vi "input.vi"(8 "error in":errorcluster, 10 "data table in":T1, 11 "OPC UA runtime in":refnum<class "OPC UA Server runtime.lvclass">) -> (0 "error out":errorcluster, 2 "data table out":T1, 3 "OPC UA runtime out":refnum<class "OPC UA Server runtime.lvclass">)   [LabVIEW 2013, in "OPC UA Server runtime.lvclass"]
doc: "Provides an interface for reading data from a module at runtime. While this interface performs no operations, a child should provide an override which may read from any open sessions, references, or interfaces."
uses:
  OPC UA Server runtime.lvclass
  <vilib>/NI/Tag Bus/table/data table.ctl
  OPC UA Server runtime.lvclass/OPC UA Server runtime.ctl
  <vilib>/NI/Tag Bus/table/data polymorphs/write one/write Boolean.vi
  <vilib>/NI/Tag Bus/table/data polymorphs/write one/write I8.vi
  <vilib>/NI/Tag Bus/table/data polymorphs/write one/write U8.vi
  <vilib>/NI/Tag Bus/table/data polymorphs/write one/write I16.vi
  <vilib>/NI/Tag Bus/table/data polymorphs/write one/write U16.vi
  <vilib>/NI/Tag Bus/table/data polymorphs/write one/write I32.vi
  <vilib>/NI/Tag Bus/table/data polymorphs/write one/write U32.vi
  <vilib>/NI/Tag Bus/table/data polymorphs/write one/write I64.vi
  <vilib>/NI/Tag Bus/table/data polymorphs/write one/write U64.vi
  <vilib>/NI/Tag Bus/table/data polymorphs/write one/write Single.vi
  <vilib>/NI/Tag Bus/table/data polymorphs/write one/write Double.vi
  <vilib>/NI/Tag Bus/table/data polymorphs/write one/write String.vi
  <vilib>/NI/Tag Bus/table/data polymorphs/write one/write Array of Boolean.vi
  <vilib>/NI/Tag Bus/table/data polymorphs/write one/write Array of I8.vi
  <vilib>/NI/Tag Bus/table/data polymorphs/write one/write Array of U8.vi
  <vilib>/NI/Tag Bus/table/data polymorphs/write one/write Array of I16.vi
  <vilib>/NI/Tag Bus/table/data polymorphs/write one/write Array of U16.vi
  <vilib>/NI/Tag Bus/table/data polymorphs/write one/write Array of I32.vi
  <vilib>/NI/Tag Bus/table/data polymorphs/write one/write Array of U32.vi
  <vilib>/NI/Tag Bus/table/data polymorphs/write one/write Array of I64.vi
  <vilib>/NI/Tag Bus/table/data polymorphs/write one/write Array of U64.vi
  <vilib>/NI/Tag Bus/table/data polymorphs/write one/write Array of Single.vi
  <vilib>/NI/Tag Bus/table/data polymorphs/write one/write Array of Double.vi
  <vilib>/NI/Tag Bus/table/data polymorphs/write one/write Array of String.vi
  <vilib>/OPCUA/server/Read Bool.vi
  <vilib>/OPCUA/server/Read SByte.vi
  <vilib>/OPCUA/server/Read Byte.vi
  <vilib>/OPCUA/server/Read Int16.vi
  <vilib>/OPCUA/server/Read UInt16.vi
  <vilib>/OPCUA/server/Read Int32.vi
  <vilib>/OPCUA/server/Read UInt32.vi
  <vilib>/OPCUA/server/Read Int64.vi
  <vilib>/OPCUA/server/Read UInt64.vi
  <vilib>/OPCUA/server/Read Float.vi
  <vilib>/OPCUA/server/Read Double.vi
  <vilib>/OPCUA/server/Read String.vi
  <vilib>/OPCUA/server/Read Date Time.vi
  <vilib>/OPCUA/server/Read Byte String.vi
  <vilib>/OPCUA/server/Read Bool Array.vi
  <vilib>/OPCUA/server/Read SByte Array.vi
  <vilib>/OPCUA/server/Read Byte Array.vi
  <vilib>/OPCUA/server/Read Int16 Array.vi
  <vilib>/OPCUA/server/Read UInt16 Array.vi
  <vilib>/OPCUA/server/Read Int32 Array.vi
  <vilib>/OPCUA/server/Read UInt32 Array.vi
  <vilib>/OPCUA/server/Read Int64 Array.vi
  <vilib>/OPCUA/server/Read UInt64 Array.vi
  <vilib>/OPCUA/server/Read Float Array.vi
  <vilib>/OPCUA/server/Read Double Array.vi
  <vilib>/OPCUA/server/Read String Array.vi
  <vilib>/OPCUA/server/Read Date Time Array.vi
  <vilib>/OPCUA/server/Read Byte String Array.vi
  <vilib>/Utility/error.llb/Error Cluster From Error Code.vi
  <vilib>/OPCUA/client/Read Bool.vi
  <vilib>/OPCUA/client/Read SByte.vi
  <vilib>/OPCUA/client/Read Byte.vi
  <vilib>/OPCUA/client/Read Int16.vi
  <vilib>/OPCUA/client/Read UInt16.vi
  <vilib>/OPCUA/client/Read Int32.vi
  <vilib>/OPCUA/client/Read UInt32.vi
  <vilib>/OPCUA/client/Read Int64.vi
  <vilib>/OPCUA/client/Read UInt64.vi
  <vilib>/OPCUA/client/Read Float.vi
  <vilib>/OPCUA/client/Read Double.vi
  <vilib>/OPCUA/client/Read String.vi
  <vilib>/OPCUA/client/Read DateTime.vi
  <vilib>/OPCUA/client/Read ByteString.vi
  <vilib>/OPCUA/client/Read Bool Array.vi
  <vilib>/OPCUA/client/Read SByte Array.vi
  <vilib>/OPCUA/client/Read Byte Array.vi
  <vilib>/OPCUA/client/Read Int16 Array.vi
  <vilib>/OPCUA/client/Read UInt16 Array.vi
  <vilib>/OPCUA/client/Read Int32 Array.vi
  <vilib>/OPCUA/client/Read UInt32 Array.vi
  <vilib>/OPCUA/client/Read Int64 Array.vi
  <vilib>/OPCUA/client/Read UInt64 Array.vi
  <vilib>/OPCUA/client/Read Float Array.vi
  <vilib>/OPCUA/client/Read Double Array.vi
  <vilib>/OPCUA/client/Read String Array.vi
  <vilib>/OPCUA/client/Read DateTime Array.vi
  <vilib>/OPCUA/client/Read ByteString Array.vi
  <vilib>/ErrorRing/Error Ring.xnode
  <vilib>/NI/Tag Bus/table/data table.lvlib
  <vilib>/opcua/NI OPC UA Client.lvlib
  <vilib>/opcua/NI OPC UA Server.lvlib
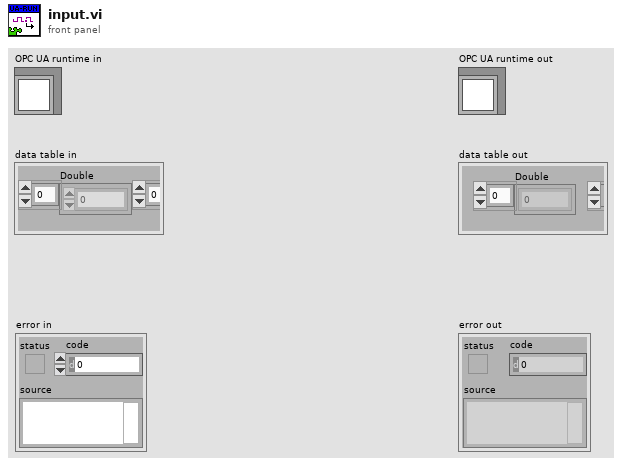
[diagram p1: front panel]
types:
  T1 = typedef "tag bus.lvlib/data table.lvlib/data table.ctl" = cluster{"Double":dbl[], "Single":sgl[], "I64":i64[], "I32":i32[], "I16":i16[], "I8":i8[], "U64":u64[], "U32":u32[], "U16":u16[], "U8":u8[], "Boolean":bool[], "String":string[], "Array of Double":cluster{"DBL Array":dbl[]}[], "Array of Single":cluster{"SGL Array":sgl[]}[], "Array of I64":cluster{"I64 Array":i64[]}[], "Array of I32":cluster{"I32 Array":i32[]}[], "Array of I16":cluster{"I16 Array":i16[]}[], "Array of I8":cluster{"I8 Array":i8[]}[], "Array of U64":cluster{"U64 Array":u64[]}[], "Array of U32":cluster{"U32 Array":u32[]}[], "Array of U16":cluster{"U16 Array":u16[]}[], "Array of U8":cluster{"U8 Array":u8[]}[], "Array of Boolean":cluster{"Boolean Array":bool[]}[], "Array of String":cluster{"String Array":string[]}[]}
  T2 = typedef "tag bus.lvlib/tag descriptor.lvclass/Data Type.ctl" = enum16{"Double", "Single", "I64", "I32", "I16", "I8", "U64", "U32", "U16", "U8", "Boolean", "String", "Array of Double", "Array of Single", "Array of I64", "Array of I32", "Array of I16", "Array of I8", "Array of U64", "Array of U32", "Array of U16", "Array of U8", "Array of Boolean", "Array of String"}
  T3 = typedef "OPC UA Server configuration.lvclass/OPC UA Data Type.ctl" = u16
  T4 = cluster{"DCAF Data Type":T2, "Index":i32, "Node Path":string, "OPC UA Data Type":T3}[]
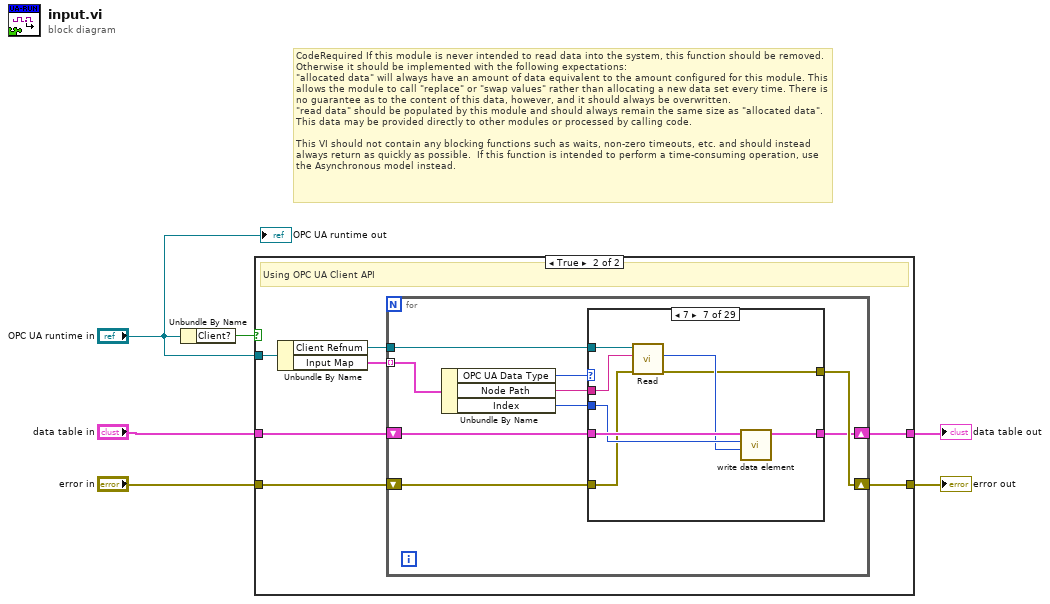
[diagram p0: block diagram]
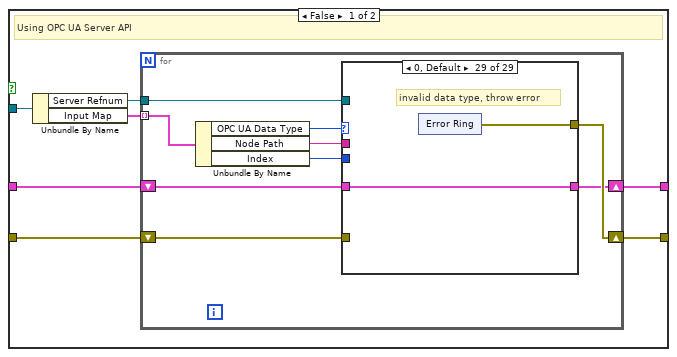
[diagram p2: hidden frame]
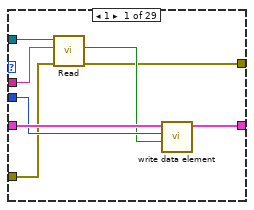
[diagram p3: hidden frame]
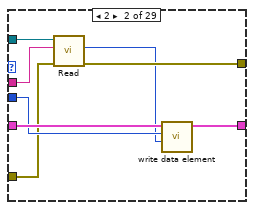
[diagram p4: hidden frame]
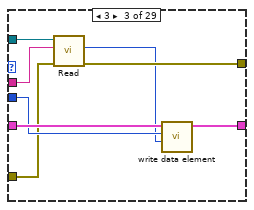
[diagram p5: hidden frame]
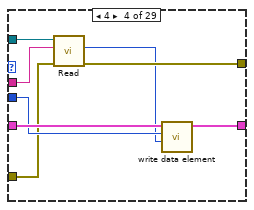
[diagram p6: hidden frame]
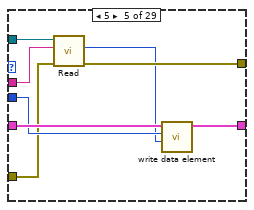
[diagram p7: hidden frame]
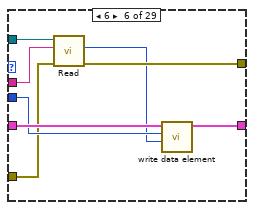
[diagram p8: hidden frame]
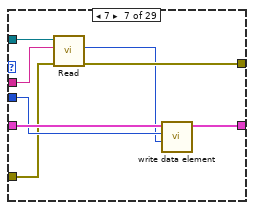
[diagram p9: hidden frame]
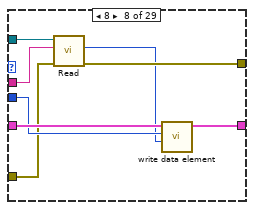
[diagram p10: hidden frame]
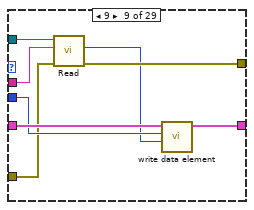
[diagram p11: hidden frame]
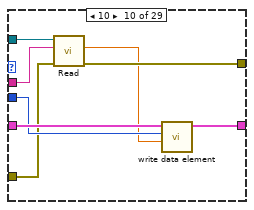
[diagram p12: hidden frame]
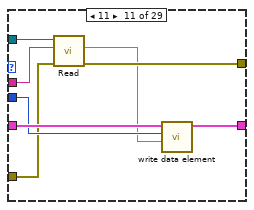
[diagram p13: hidden frame]
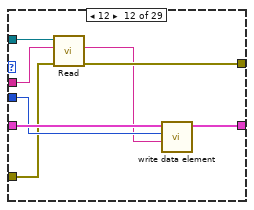
[diagram p14: hidden frame]
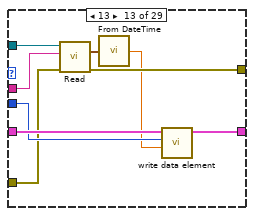
[diagram p15: hidden frame]
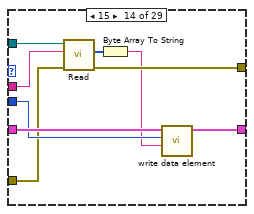
[diagram p16: hidden frame]
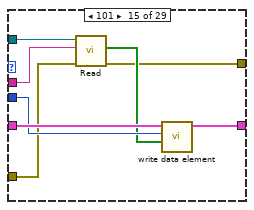
[diagram p17: hidden frame]
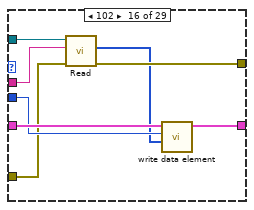
[diagram p18: hidden frame]
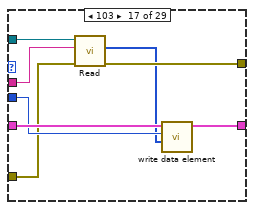
[diagram p19: hidden frame]
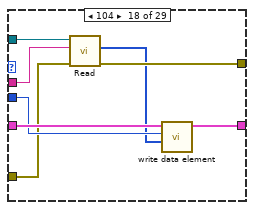
[diagram p20: hidden frame]
diagram:
  # "CodeRequired If this module is never intended to read data into the system, this function should be removed. Otherwise it should be implemented with the following expectations:\n\"allocated data\" will always have an amount of data equivalent to the amount configured for this module. This allows the module to call \"replace\" or \"swap values\" rather than allocating a new data set every time. There is no guarantee as to the content of this data, however, and it should always be overwritten.\n\"read data\" should be populated by this module and should always remain the same size as \"allocated data\". This data may be provided directly to other modules or processed by calling code.\n\nThis VI should not contain any blocking functions such as waits, non-zero timeouts, etc. and should instead always return as quickly as possible.  If this function is intended to perform a time-consuming operation, use the Asynchronous model instead."
  n1 = Unbundle By Name("OPC UA runtime in") -> ("Client?"=w6:bool)
  n2 = case shown="True" w6 {
    tunnel: "OPC UA runtime in" -> [w13 w266]
    tunnel: "data table in" -> [w9 w263]
    tunnel: "error in" -> [w8 w262]
    tunnel: [w10 w261] -> w2
    tunnel: [w7 w260] -> w1
    frame False {
      # "Using OPC UA Server API"
      n3 = Unbundle By Name(w13) -> ("Server Refnum"=w11:refnum<k21>, "Input Map"=w12:T4)
      n4 = for {
        tunnel: w11 -> [w18]
        tunnel: w12 -> [w22] mode=indexing
        shift-right: [w15] -> w7
        shift-left: w8 -> [w16]
        shift-right: [w14] -> w10
        shift-left: w9 -> [w17]
        n5 = Unbundle By Name(w22) -> ("OPC UA Data Type"=w21:T3, "Node Path"=w20:string, "Index"=w19:i32)
        n6 = case shown="0, Default" w21 {
          tunnel: w20 -> [w29 w37 w45 w53 w61 w69 w77 w85 w93 w101 w109 w117 w126 w135 w144 w152 w160 w168 w176 w184 w192 w200 w208 w216 w224 w232 w241 w249 _]
          tunnel: w19 -> [w27 w35 w43 w51 w59 w67 w75 w83 w91 w99 w107 w115 w124 w133 w142 w150 w158 w166 w174 w182 w190 w198 w206 w214 w222 w230 w239 w247 _]
          tunnel: w18 -> [w30 w38 w46 w54 w62 w70 w78 w86 w94 w102 w110 w118 w127 w136 w137 w146 w153 w162 w170 w178 w186 w194 w202 w210 w218 w225 w234 w250 _]
          tunnel: w17 -> [w28 w36 w44 w52 w60 w68 w76 w84 w92 w100 w108 w116 w125 w134 w143 w151 w159 w167 w175 w183 w191 w199 w207 w215 w223 w231 w240 w248 w254]
          tunnel: w16 -> [w25 w34 w42 w50 w58 w66 w74 w82 w90 w98 w106 w114 w123 w132 w140 w149 w157 w165 w173 w181 w189 w197 w205 w213 w221 w228 w238 w246 _]
          tunnel: [w24 w33 w41 w49 w57 w65 w73 w81 w89 w97 w105 w113 w122 w131 w139 w148 w156 w164 w172 w180 w188 w196 w204 w212 w220 w227 w237 w245 w253] -> w15
          tunnel: [w23 w32 w40 w48 w56 w64 w72 w80 w88 w96 w104 w112 w121 w130 w138 w147 w155 w163 w171 w179 w187 w195 w203 w211 w219 w226 w236 w244 w254] -> w14
          frame 1 {
            n7 = call-poly <vilib>:"Read.vi"("error in (no error)"=w25, "node path"=w29, "OPC UA server refnum in"=w30) -> ("error out"=w24:errorcluster, "value"=w26:bool)  [unwired: 4 in, 3 out]
            n8 = call-poly <vilib>:"write data element.vi"("value"=w26, "index"=w27, "data table in"=w28) -> ("data table out"=w23:T1)  [unwired: 8 in]
          }
          frame 2 {
            n9 = call-poly <vilib>:"Read.vi"("error in (no error)"=w34, "node path"=w37, "OPC UA server refnum in"=w38) -> ("error out"=w33:errorcluster, "value"=w31:i8)  [unwired: 4 in, 3 out]
            n10 = call-poly <vilib>:"write data element.vi"("value"=w31, "index"=w35, "data table in"=w36) -> ("data table out"=w32:T1)  [unwired: 8 in]
          }
          frame 3 {
            n11 = call-poly <vilib>:"Read.vi"("error in (no error)"=w42, "node path"=w45, "OPC UA server refnum in"=w46) -> ("error out"=w41:errorcluster, "value"=w39:u8)  [unwired: 4 in, 3 out]
            n12 = call-poly <vilib>:"write data element.vi"("value"=w39, "index"=w43, "data table in"=w44) -> ("data table out"=w40:T1)  [unwired: 8 in]
          }
          frame 4 {
            n13 = call-poly <vilib>:"Read.vi"("error in (no error)"=w50, "node path"=w53, "OPC UA server refnum in"=w54) -> ("error out"=w49:errorcluster, "value"=w47:i16)  [unwired: 4 in, 3 out]
            n14 = call-poly <vilib>:"write data element.vi"("value"=w47, "index"=w51, "data table in"=w52) -> ("data table out"=w48:T1)  [unwired: 8 in]
          }
          frame 5 {
            n15 = call-poly <vilib>:"Read.vi"("error in (no error)"=w58, "node path"=w61, "OPC UA server refnum in"=w62) -> ("error out"=w57:errorcluster, "value"=w55:u16)  [unwired: 4 in, 3 out]
            n16 = call-poly <vilib>:"write data element.vi"("value"=w55, "index"=w59, "data table in"=w60) -> ("data table out"=w56:T1)  [unwired: 8 in]
          }
          frame 6 {
            n17 = call-poly <vilib>:"Read.vi"("error in (no error)"=w66, "node path"=w69, "OPC UA server refnum in"=w70) -> ("error out"=w65:errorcluster, "value"=w63:i32)  [unwired: 4 in, 3 out]
            n18 = call-poly <vilib>:"write data element.vi"("value"=w63, "index"=w67, "data table in"=w68) -> ("data table out"=w64:T1)  [unwired: 8 in]
          }
          frame 7 {
            n19 = call-poly <vilib>:"Read.vi"("error in (no error)"=w74, "node path"=w77, "OPC UA server refnum in"=w78) -> ("error out"=w73:errorcluster, "value"=w71:u32)  [unwired: 4 in, 3 out]
            n20 = call-poly <vilib>:"write data element.vi"("value"=w71, "index"=w75, "data table in"=w76) -> ("data table out"=w72:T1)  [unwired: 8 in]
          }
          frame 8 {
            n21 = call-poly <vilib>:"Read.vi"("error in (no error)"=w82, "node path"=w85, "OPC UA server refnum in"=w86) -> ("error out"=w81:errorcluster, "value"=w79:i64)  [unwired: 4 in, 3 out]
            n22 = call-poly <vilib>:"write data element.vi"("value"=w79, "index"=w83, "data table in"=w84) -> ("data table out"=w80:T1)  [unwired: 8 in]
          }
          frame 9 {
            n23 = call-poly <vilib>:"Read.vi"("error in (no error)"=w90, "node path"=w93, "OPC UA server refnum in"=w94) -> ("error out"=w89:errorcluster, "value"=w87:u64)  [unwired: 4 in, 3 out]
            n24 = call-poly <vilib>:"write data element.vi"("value"=w87, "index"=w91, "data table in"=w92) -> ("data table out"=w88:T1)  [unwired: 8 in]
          }
          frame 10 {
            n25 = call-poly <vilib>:"Read.vi"("error in (no error)"=w98, "node path"=w101, "OPC UA server refnum in"=w102) -> ("error out"=w97:errorcluster, "value"=w95:sgl)  [unwired: 4 in, 3 out]
            n26 = call-poly <vilib>:"write data element.vi"("value"=w95, "index"=w99, "data table in"=w100) -> ("data table out"=w96:T1)  [unwired: 8 in]
          }
          frame 11 {
            n27 = call-poly <vilib>:"Read.vi"("error in (no error)"=w106, "node path"=w109, "OPC UA server refnum in"=w110) -> ("error out"=w105:errorcluster, "value"=w103:dbl)  [unwired: 4 in, 3 out]
            n28 = call-poly <vilib>:"write data element.vi"("value"=w103, "index"=w107, "data table in"=w108) -> ("data table out"=w104:T1)  [unwired: 8 in]
          }
          frame 12 {
            n29 = call-poly <vilib>:"Read.vi"("error in (no error)"=w114, "node path"=w117, "OPC UA server refnum in"=w118) -> ("error out"=w113:errorcluster, "value"=w111:string)  [unwired: 4 in, 3 out]
            n30 = call-poly <vilib>:"write data element.vi"("value"=w111, "index"=w115, "data table in"=w116) -> ("data table out"=w112:T1)  [unwired: 8 in]
          }
          frame 13 {
            n31 = call-poly <vilib>:"Read.vi"("error in (error in)"=w123, "node path"=w126, "OPC UA server refnum in"=w127) -> ("error out"=w122:errorcluster, "timestamp"=w120:timestamp)  [unwired: 4 in, 3 out]
            n32 = call "From DateTime.vi"("DateTime"=w120) -> ("Formatted DateTime"=w119:dbl)
            n33 = call-poly <vilib>:"write data element.vi"("value"=w119, "index"=w124, "data table in"=w125) -> ("data table out"=w121:T1)  [unwired: 8 in]
          }
          frame 15 {
            n34 = call-poly <vilib>:"Read.vi"("error in (no error)"=w132, "node path"=w135, "OPC UA server refnum in"=w136) -> ("error out"=w131:errorcluster, "value"=w128:u8[])  [unwired: 4 in, 3 out]
            n35 = Byte Array To String(unsigned byte array=w128) -> (string=w129:string)
            n36 = call-poly <vilib>:"write data element.vi"("value"=w129, "index"=w133, "data table in"=w134) -> ("data table out"=w130:T1)  [unwired: 8 in]
          }
          frame 101 {
            n37 = call-poly <vilib>:"Read.vi"("error in (no error)"=w140, "node path"=w144, "OPC UA server refnum in"=w137) -> ("error out"=w139:errorcluster, "value"=w141:bool[])  [unwired: 4 in, 3 out]
            n38 = call-poly <vilib>:"write data element.vi"("value"=w141, "index"=w142, "data table in"=w143) -> ("data table out"=w138:T1)  [unwired: 8 in]
          }
          frame 102 {
            n39 = call-poly <vilib>:"Read.vi"("error in (no error)"=w149, "node path"=w152, "OPC UA server refnum in"=w146) -> ("error out"=w148:errorcluster, "value"=w145:i8[])  [unwired: 4 in, 3 out]
            n40 = call-poly <vilib>:"write data element.vi"("value"=w145, "index"=w150, "data table in"=w151) -> ("data table out"=w147:T1)  [unwired: 8 in]
          }
          frame 103 {
            n41 = call-poly <vilib>:"Read.vi"("error in (no error)"=w157, "node path"=w160, "OPC UA server refnum in"=w153) -> ("error out"=w156:errorcluster, "value"=w154:u8[])  [unwired: 4 in, 3 out]
            n42 = call-poly <vilib>:"write data element.vi"("value"=w154, "index"=w158, "data table in"=w159) -> ("data table out"=w155:T1)  [unwired: 8 in]
          }
          frame 104 {
            n43 = call-poly <vilib>:"Read.vi"("error in (no error)"=w165, "node path"=w168, "OPC UA server refnum in"=w162) -> ("error out"=w164:errorcluster, "value"=w161:i16[])  [unwired: 4 in, 3 out]
            n44 = call-poly <vilib>:"write data element.vi"("value"=w161, "index"=w166, "data table in"=w167) -> ("data table out"=w163:T1)  [unwired: 8 in]
          }
          frame 105 {
            n45 = call-poly <vilib>:"Read.vi"("error in (no error)"=w173, "node path"=w176, "OPC UA server refnum in"=w170) -> ("error out"=w172:errorcluster, "value"=w169:u16[])  [unwired: 4 in, 3 out]
            n46 = call-poly <vilib>:"write data element.vi"("value"=w169, "index"=w174, "data table in"=w175) -> ("data table out"=w171:T1)  [unwired: 8 in]
          }
          frame 106 {
            n47 = call-poly <vilib>:"Read.vi"("error in (no error)"=w181, "node path"=w184, "OPC UA server refnum in"=w178) -> ("error out"=w180:errorcluster, "value"=w177:i32[])  [unwired: 4 in, 3 out]
            n48 = call-poly <vilib>:"write data element.vi"("value"=w177, "index"=w182, "data table in"=w183) -> ("data table out"=w179:T1)  [unwired: 8 in]
          }
          frame 107 {
            n49 = call-poly <vilib>:"Read.vi"("error in (no error)"=w189, "node path"=w192, "OPC UA server refnum in"=w186) -> ("error out"=w188:errorcluster, "value"=w185:u32[])  [unwired: 4 in, 3 out]
            n50 = call-poly <vilib>:"write data element.vi"("value"=w185, "index"=w190, "data table in"=w191) -> ("data table out"=w187:T1)  [unwired: 8 in]
          }
          frame 108 {
            n51 = call-poly <vilib>:"Read.vi"("error in (no error)"=w197, "node path"=w200, "OPC UA server refnum in"=w194) -> ("error out"=w196:errorcluster, "value"=w193:i64[])  [unwired: 4 in, 3 out]
            n52 = call-poly <vilib>:"write data element.vi"("value"=w193, "index"=w198, "data table in"=w199) -> ("data table out"=w195:T1)  [unwired: 8 in]
          }
          frame 109 {
            n53 = call-poly <vilib>:"Read.vi"("error in (no error)"=w205, "node path"=w208, "OPC UA server refnum in"=w202) -> ("error out"=w204:errorcluster, "value"=w201:u64[])  [unwired: 4 in, 3 out]
            n54 = call-poly <vilib>:"write data element.vi"("value"=w201, "index"=w206, "data table in"=w207) -> ("data table out"=w203:T1)  [unwired: 8 in]
          }
          frame 110 {
            n55 = call-poly <vilib>:"Read.vi"("error in (no error)"=w213, "node path"=w216, "OPC UA server refnum in"=w210) -> ("error out"=w212:errorcluster, "value"=w209:sgl[])  [unwired: 4 in, 3 out]
            n56 = call-poly <vilib>:"write data element.vi"("value"=w209, "index"=w214, "data table in"=w215) -> ("data table out"=w211:T1)  [unwired: 8 in]
          }
          frame 111 {
            n57 = call-poly <vilib>:"Read.vi"("error in (no error)"=w221, "node path"=w224, "OPC UA server refnum in"=w218) -> ("error out"=w220:errorcluster, "value"=w217:dbl[])  [unwired: 4 in, 3 out]
            n58 = call-poly <vilib>:"write data element.vi"("value"=w217, "index"=w222, "data table in"=w223) -> ("data table out"=w219:T1)  [unwired: 8 in]
          }
          frame 112 {
            n59 = call-poly <vilib>:"Read.vi"("error in (no error)"=w228, "node path"=w232, "OPC UA server refnum in"=w225) -> ("error out"=w227:errorcluster, "value"=w229:string[])  [unwired: 4 in, 3 out]
            n60 = call-poly <vilib>:"write data element.vi"("value"=w229, "index"=w230, "data table in"=w231) -> ("data table out"=w226:T1)  [unwired: 8 in]
          }
          frame 113 {
            n61 = call-poly <vilib>:"Read.vi"("error in (no error)"=w238, "node path"=w241, "OPC UA server refnum in"=w234) -> ("error out"=w237:errorcluster, "value"=w233:timestamp[])  [unwired: 4 in, 3 out]
            n62 = call "From DateTime Array.vi"("DateTime Array"=w233) -> ("Formatted DateTime Array"=w235:dbl[])
            n63 = call-poly <vilib>:"write data element.vi"("value"=w235, "index"=w239, "data table in"=w240) -> ("data table out"=w236:T1)  [unwired: 8 in]
          }
          frame 115 {
            n64 = call-poly <vilib>:"Read.vi"("error in (no error)"=w246, "node path"=w249, "OPC UA server refnum in"=w250) -> ("error out"=w245:errorcluster, "value"=w242:u8[][])  [unwired: 4 in, 3 out]
            n65 = for {
              tunnel: [w252] -> w243 mode=indexing
              tunnel: w242 -> [w251] mode=indexing
              n66 = Byte Array To String(unsigned byte array=w251) -> (string=w252:string)
            }
            n67 = call-poly <vilib>:"write data element.vi"("value"=w243, "index"=w247, "data table in"=w248) -> ("data table out"=w244:T1)  [unwired: 8 in]
          }
          frame 0, Default {
            # "invalid data type, throw error"
            n68 = xnode "Error Ring"() -> ("error out"=w253:errorcluster)
          }
        }
      }
    }
    frame True {
      # "Using OPC UA Client API"
      n69 = Unbundle By Name(w266) -> ("Client Refnum"=w265:refnum<k21>, "Input Map"=w264:T4)
      n70 = for {
        tunnel: w265 -> [w271]
        tunnel: w264 -> [w275] mode=indexing
        shift-right: [w268] -> w260
        shift-left: w262 -> [w269]
        shift-right: [w267] -> w261
        shift-left: w263 -> [w270]
        n71 = Unbundle By Name(w275) -> ("OPC UA Data Type"=w274:T3, "Node Path"=w273:string, "Index"=w272:i32)
        n72 = case shown="7" w274 {
          tunnel: w273 -> [w282 w290 w298 w306 w314 w322 w330 w338 w346 w354 w362 w370 w379 w388 w396 w404 w412 w420 w428 w436 w444 w452 w460 w468 w476 w484 w493 w502 _]
          tunnel: w272 -> [w280 w288 w296 w304 w312 w320 w328 w336 w344 w352 w360 w368 w377 w386 w394 w402 w410 w418 w426 w434 w442 w450 w458 w466 w474 w482 w491 w500 _]
          tunnel: w271 -> [w283 w291 w299 w307 w315 w323 w331 w339 w347 w355 w363 w371 w380 w389 w397 w405 w413 w421 w429 w437 w445 w453 w461 w469 w477 w485 w494 w503 _]
          tunnel: w270 -> [w281 w289 w297 w305 w313 w321 w329 w337 w345 w353 w361 w369 w378 w387 w395 w403 w411 w419 w427 w435 w443 w451 w459 w467 w475 w483 w492 w501 w506]
          tunnel: w269 -> [w278 w286 w294 w302 w310 w318 w326 w334 w342 w350 w358 w366 w376 w385 w392 w400 w408 w416 w424 w432 w440 w448 w456 w464 w472 w480 w490 w499 _]
          tunnel: [w277 w285 w293 w301 w309 w317 w325 w333 w341 w349 w357 w365 w375 w384 w391 w399 w407 w415 w423 w431 w439 w447 w455 w463 w471 w479 w489 w498 w507] -> w268
          tunnel: [w276 w284 w292 w300 w308 w316 w324 w332 w340 w348 w356 w364 w374 w383 w390 w398 w406 w414 w422 w430 w438 w446 w454 w462 w470 w478 w488 w497 w506] -> w267
          frame 1 {
            n73 = call-poly <vilib>:"Read.vi"("error in (no error)"=w278, "node path"=w282, "OPC UA client refnum in"=w283) -> ("error out"=w277:errorcluster, "value"=w279:bool)  [unwired: 4 in, 3 out]
            n74 = call-poly <vilib>:"write data element.vi"("value"=w279, "index"=w280, "data table in"=w281) -> ("data table out"=w276:T1)  [unwired: 8 in]
          }
          frame 2 {
            n75 = call-poly <vilib>:"Read.vi"("error in (no error)"=w286, "node path"=w290, "OPC UA client refnum in"=w291) -> ("error out"=w285:errorcluster, "value"=w287:i8)  [unwired: 4 in, 3 out]
            n76 = call-poly <vilib>:"write data element.vi"("value"=w287, "index"=w288, "data table in"=w289) -> ("data table out"=w284:T1)  [unwired: 8 in]
          }
          frame 3 {
            n77 = call-poly <vilib>:"Read.vi"("error in (no error)"=w294, "node path"=w298, "OPC UA client refnum in"=w299) -> ("error out"=w293:errorcluster, "value"=w295:u8)  [unwired: 4 in, 3 out]
            n78 = call-poly <vilib>:"write data element.vi"("value"=w295, "index"=w296, "data table in"=w297) -> ("data table out"=w292:T1)  [unwired: 8 in]
          }
          frame 4 {
            n79 = call-poly <vilib>:"Read.vi"("error in (no error)"=w302, "node path"=w306, "OPC UA client refnum in"=w307) -> ("error out"=w301:errorcluster, "value"=w303:i16)  [unwired: 4 in, 3 out]
            n80 = call-poly <vilib>:"write data element.vi"("value"=w303, "index"=w304, "data table in"=w305) -> ("data table out"=w300:T1)  [unwired: 8 in]
          }
          frame 5 {
            n81 = call-poly <vilib>:"Read.vi"("error in (no error)"=w310, "node path"=w314, "OPC UA client refnum in"=w315) -> ("error out"=w309:errorcluster, "value"=w311:u16)  [unwired: 4 in, 3 out]
            n82 = call-poly <vilib>:"write data element.vi"("value"=w311, "index"=w312, "data table in"=w313) -> ("data table out"=w308:T1)  [unwired: 8 in]
          }
          frame 6 {
            n83 = call-poly <vilib>:"Read.vi"("error in (no error)"=w318, "node path"=w322, "OPC UA client refnum in"=w323) -> ("error out"=w317:errorcluster, "value"=w319:i32)  [unwired: 4 in, 3 out]
            n84 = call-poly <vilib>:"write data element.vi"("value"=w319, "index"=w320, "data table in"=w321) -> ("data table out"=w316:T1)  [unwired: 8 in]
          }
          frame 7 {
            n85 = call-poly <vilib>:"Read.vi"("error in (no error)"=w326, "node path"=w330, "OPC UA client refnum in"=w331) -> ("error out"=w325:errorcluster, "value"=w327:u32)  [unwired: 4 in, 3 out]
            n86 = call-poly <vilib>:"write data element.vi"("value"=w327, "index"=w328, "data table in"=w329) -> ("data table out"=w324:T1)  [unwired: 8 in]
          }
          frame 8 {
            n87 = call-poly <vilib>:"Read.vi"("error in (no error)"=w334, "node path"=w338, "OPC UA client refnum in"=w339) -> ("error out"=w333:errorcluster, "value"=w335:i64)  [unwired: 4 in, 3 out]
            n88 = call-poly <vilib>:"write data element.vi"("value"=w335, "index"=w336, "data table in"=w337) -> ("data table out"=w332:T1)  [unwired: 8 in]
          }
          frame 9 {
            n89 = call-poly <vilib>:"Read.vi"("error in (no error)"=w342, "node path"=w346, "OPC UA client refnum in"=w347) -> ("error out"=w341:errorcluster, "value"=w343:u64)  [unwired: 4 in, 3 out]
            n90 = call-poly <vilib>:"write data element.vi"("value"=w343, "index"=w344, "data table in"=w345) -> ("data table out"=w340:T1)  [unwired: 8 in]
          }
          frame 10 {
            n91 = call-poly <vilib>:"Read.vi"("error in (no error)"=w350, "node path"=w354, "OPC UA client refnum in"=w355) -> ("error out"=w349:errorcluster, "value"=w351:sgl)  [unwired: 4 in, 3 out]
            n92 = call-poly <vilib>:"write data element.vi"("value"=w351, "index"=w352, "data table in"=w353) -> ("data table out"=w348:T1)  [unwired: 8 in]
          }
          frame 11 {
            n93 = call-poly <vilib>:"Read.vi"("error in (no error)"=w358, "node path"=w362, "OPC UA client refnum in"=w363) -> ("error out"=w357:errorcluster, "value"=w359:dbl)  [unwired: 4 in, 3 out]
            n94 = call-poly <vilib>:"write data element.vi"("value"=w359, "index"=w360, "data table in"=w361) -> ("data table out"=w356:T1)  [unwired: 8 in]
          }
          frame 12 {
            n95 = call-poly <vilib>:"Read.vi"("error in (no error)"=w366, "node path"=w370, "OPC UA client refnum in"=w371) -> ("error out"=w365:errorcluster, "value"=w367:string)  [unwired: 4 in, 3 out]
            n96 = call-poly <vilib>:"write data element.vi"("value"=w367, "index"=w368, "data table in"=w369) -> ("data table out"=w364:T1)  [unwired: 8 in]
          }
          frame 13 {
            n97 = call-poly <vilib>:"Read.vi"("error in (no error)"=w376, "node path"=w379, "OPC UA client refnum in"=w380) -> ("error out"=w375:errorcluster, "value"=w373:timestamp)  [unwired: 4 in, 3 out]
            n98 = call "From DateTime.vi"("DateTime"=w373) -> ("Formatted DateTime"=w372:dbl)
            n99 = call-poly <vilib>:"write data element.vi"("value"=w372, "index"=w377, "data table in"=w378) -> ("data table out"=w374:T1)  [unwired: 8 in]
          }
          frame 15 {
            n100 = call-poly <vilib>:"Read.vi"("error in (no error)"=w385, "node path"=w388, "OPC UA client refnum in"=w389) -> ("error out"=w384:errorcluster, "value"=w382:u8[])  [unwired: 4 in, 3 out]
            n101 = Byte Array To String(unsigned byte array=w382) -> (string=w381:string)
            n102 = call-poly <vilib>:"write data element.vi"("value"=w381, "index"=w386, "data table in"=w387) -> ("data table out"=w383:T1)  [unwired: 8 in]
          }
          frame 101 {
            n103 = call-poly <vilib>:"Read.vi"("error in (no error)"=w392, "node path"=w396, "OPC UA client refnum in"=w397) -> ("error out"=w391:errorcluster, "value"=w393:bool[])  [unwired: 4 in, 3 out]
            n104 = call-poly <vilib>:"write data element.vi"("value"=w393, "index"=w394, "data table in"=w395) -> ("data table out"=w390:T1)  [unwired: 8 in]
          }
          frame 102 {
            n105 = call-poly <vilib>:"Read.vi"("error in (no error)"=w400, "node path"=w404, "OPC UA client refnum in"=w405) -> ("error out"=w399:errorcluster, "value"=w401:i8[])  [unwired: 4 in, 3 out]
            n106 = call-poly <vilib>:"write data element.vi"("value"=w401, "index"=w402, "data table in"=w403) -> ("data table out"=w398:T1)  [unwired: 8 in]
          }
          frame 103 {
            n107 = call-poly <vilib>:"Read.vi"("error in (no error)"=w408, "node path"=w412, "OPC UA client refnum in"=w413) -> ("error out"=w407:errorcluster, "value"=w409:u8[])  [unwired: 4 in, 3 out]
            n108 = call-poly <vilib>:"write data element.vi"("value"=w409, "index"=w410, "data table in"=w411) -> ("data table out"=w406:T1)  [unwired: 8 in]
          }
          frame 104 {
            n109 = call-poly <vilib>:"Read.vi"("error in (no error)"=w416, "node path"=w420, "OPC UA client refnum in"=w421) -> ("error out"=w415:errorcluster, "value"=w417:i16[])  [unwired: 4 in, 3 out]
            n110 = call-poly <vilib>:"write data element.vi"("value"=w417, "index"=w418, "data table in"=w419) -> ("data table out"=w414:T1)  [unwired: 8 in]
          }
          frame 105 {
            n111 = call-poly <vilib>:"Read.vi"("error in (no error)"=w424, "node path"=w428, "OPC UA client refnum in"=w429) -> ("error out"=w423:errorcluster, "value"=w425:u16[])  [unwired: 4 in, 3 out]
            n112 = call-poly <vilib>:"write data element.vi"("value"=w425, "index"=w426, "data table in"=w427) -> ("data table out"=w422:T1)  [unwired: 8 in]
          }
          frame 106 {
            n113 = call-poly <vilib>:"Read.vi"("error in (no error)"=w432, "node path"=w436, "OPC UA client refnum in"=w437) -> ("error out"=w431:errorcluster, "value"=w433:i32[])  [unwired: 4 in, 3 out]
            n114 = call-poly <vilib>:"write data element.vi"("value"=w433, "index"=w434, "data table in"=w435) -> ("data table out"=w430:T1)  [unwired: 8 in]
          }
          frame 107 {
            n115 = call-poly <vilib>:"Read.vi"("error in (no error)"=w440, "node path"=w444, "OPC UA client refnum in"=w445) -> ("error out"=w439:errorcluster, "value"=w441:u32[])  [unwired: 4 in, 3 out]
            n116 = call-poly <vilib>:"write data element.vi"("value"=w441, "index"=w442, "data table in"=w443) -> ("data table out"=w438:T1)  [unwired: 8 in]
          }
          frame 108 {
            n117 = call-poly <vilib>:"Read.vi"("error in (no error)"=w448, "node path"=w452, "OPC UA client refnum in"=w453) -> ("error out"=w447:errorcluster, "value"=w449:i64[])  [unwired: 4 in, 3 out]
            n118 = call-poly <vilib>:"write data element.vi"("value"=w449, "index"=w450, "data table in"=w451) -> ("data table out"=w446:T1)  [unwired: 8 in]
          }
          frame 109 {
            n119 = call-poly <vilib>:"Read.vi"("error in (no error)"=w456, "node path"=w460, "OPC UA client refnum in"=w461) -> ("error out"=w455:errorcluster, "value"=w457:u64[])  [unwired: 4 in, 3 out]
            n120 = call-poly <vilib>:"write data element.vi"("value"=w457, "index"=w458, "data table in"=w459) -> ("data table out"=w454:T1)  [unwired: 8 in]
          }
          frame 110 {
            n121 = call-poly <vilib>:"Read.vi"("error in (no error)"=w464, "node path"=w468, "OPC UA client refnum in"=w469) -> ("error out"=w463:errorcluster, "value"=w465:sgl[])  [unwired: 4 in, 3 out]
            n122 = call-poly <vilib>:"write data element.vi"("value"=w465, "index"=w466, "data table in"=w467) -> ("data table out"=w462:T1)  [unwired: 8 in]
          }
          frame 111 {
            n123 = call-poly <vilib>:"Read.vi"("error in (no error)"=w472, "node path"=w476, "OPC UA client refnum in"=w477) -> ("error out"=w471:errorcluster, "value"=w473:dbl[])  [unwired: 4 in, 3 out]
            n124 = call-poly <vilib>:"write data element.vi"("value"=w473, "index"=w474, "data table in"=w475) -> ("data table out"=w470:T1)  [unwired: 8 in]
          }
          frame 112 {
            n125 = call-poly <vilib>:"Read.vi"("error in (no error)"=w480, "node path"=w484, "OPC UA client refnum in"=w485) -> ("error out"=w479:errorcluster, "value"=w481:string[])  [unwired: 4 in, 3 out]
            n126 = call-poly <vilib>:"write data element.vi"("value"=w481, "index"=w482, "data table in"=w483) -> ("data table out"=w478:T1)  [unwired: 8 in]
          }
          frame 113 {
            n127 = call-poly <vilib>:"Read.vi"("error in (no error)"=w490, "node path"=w493, "OPC UA client refnum in"=w494) -> ("error out"=w489:errorcluster, "value"=w487:timestamp[])  [unwired: 4 in, 3 out]
            n128 = call "From DateTime Array.vi"("DateTime Array"=w487) -> ("Formatted DateTime Array"=w486:dbl[])
            n129 = call-poly <vilib>:"write data element.vi"("value"=w486, "index"=w491, "data table in"=w492) -> ("data table out"=w488:T1)  [unwired: 8 in]
          }
          frame 115 {
            n130 = call-poly <vilib>:"Read.vi"("error in (no error)"=w499, "node path"=w502, "OPC UA client refnum in"=w503) -> ("error out"=w498:errorcluster, "value"=w496:u8[][])  [unwired: 4 in, 3 out]
            n131 = for {
              tunnel: w496 -> [w505] mode=indexing
              tunnel: [w504] -> w495 mode=indexing
              n132 = Byte Array To String(unsigned byte array=w505) -> (string=w504:string)
            }
            n133 = call-poly <vilib>:"write data element.vi"("value"=w495, "index"=w500, "data table in"=w501) -> ("data table out"=w497:T1)  [unwired: 8 in]
          }
          frame 0, Default {
            # "invalid data type, throw error"
            n134 = xnode "Error Ring"() -> ("error out"=w507:errorcluster)
          }
        }
      }
    }
  }
  "error out" <- w1
  "data table out" <- w2
  "OPC UA runtime out" <- "OPC UA runtime in"
